vi "Send Command.vi"(8 "error in (no error)":errorcluster caption="entrée d'erreur (pas d'erreur)", 9 "Data":variant, 10 "Commands":T1="CONTROL:CHECKButtonALLON", 11 "Control en entrée":refnum<class "Control-Server.lvclass">) -> (0 "error out":errorcluster caption="sortie d'erreur", 3 "Control en sortie":refnum<class "Control-Server.lvclass">)   [LabVIEW 2018, in "Control-Server.lvclass"]
uses:
  Control-Server.lvclass
  C:/Users/Sergey Denisov/Documents/REPS/TRANCON/Classes/GeneralFunctionality/GeneralFunctionality.lvclass
  dependecies/ControlsVIs/Clusters-def/SERVER-Commands.ctl
  dependecies/ControlsVIs/Clusters-def/Message types.ctl
  Message/Message.lvclass
  GeneralFunctionality/GeneralFunctionality.lvclass
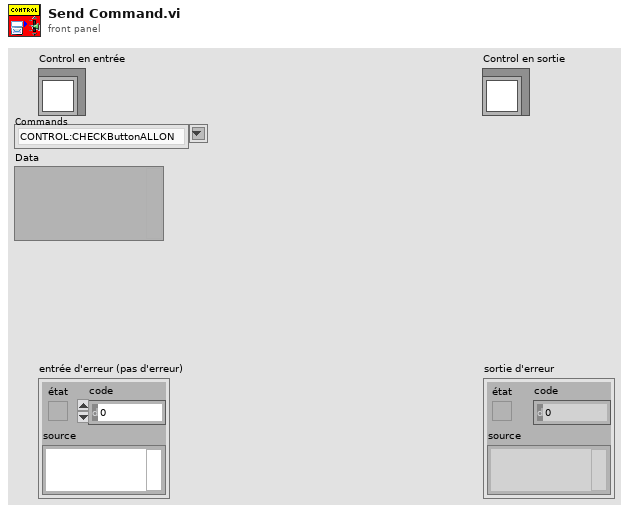
[diagram p1: front panel]
types:
  T1 = typedef "Control-Server.lvclass/SERVER-Commands.ctl" = string
  T2 = typedef "Message types.ctl" = string
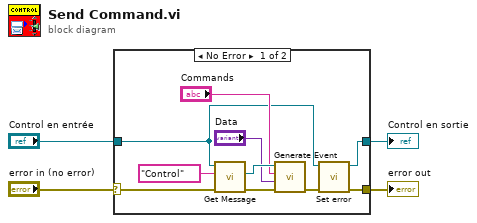
[diagram p0: block diagram]
diagram:
  n1 = case shown="No Error" "error in (no error)" {
    selector: "error in (no error)" -> [w12 w16]
    tunnel: [w5 w16] -> w3
    tunnel: [w7 w15] -> w1
    tunnel: "Control en entrée" -> [w8 w15]
    frame No Error {
      n2 = call "Get Message.vi"("error in (no error)"=w12, "Message type"=T2 "Control", "GeneralFunctionality en entrée"=w8) -> ("error out"=w13:errorcluster, "Message.lvclass"=w14:refnum<class "Message.lvclass">)  [unwired: 6 in, 1 out]
      n3 = call "Generate Event.vi"("error in (no error)"=w13, "Data"="Data", "Command"="Commands", "Message en entrée"=w14) -> ("error out"=w6:errorcluster)  [unwired: 6 in, 1 out]
      n4 = call "Set error.vi"("error in (no error)"=w6, "Control-Server in"=w8) -> ("error out"=w5:errorcluster, "Control-Server out"=w7:refnum<class "Control-Server.lvclass">)  [unwired: 8 in]
    }
    frame Error {
    }
  }
  "error out" <- w3
  "Control en sortie" <- w1
